vi "布尔与U8之间转换.vi"() -> ()   [LabVIEW 2023]
doc: "本VI是为《我和LabVIEW》一书编写的示例。\n关于本书的介绍请参考网页：\nhttp://ruanqizhen.spaces.live.com/blog/cns!5852D4F797C53FB6!4310.entry"
panel:
  out "*(类型 *) &x 2":u8
  out "*(类型 *) &x":bool
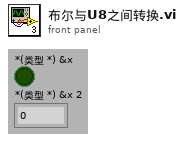
[diagram p1: front panel]
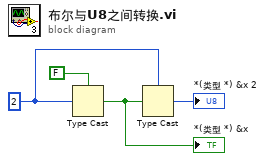
[diagram p0: block diagram]
diagram:
  w2 = u8 2 ("数值")
  n1 = Type Cast(type=FALSE, x=w2) -> (*(type *) &x=w3:bool)
  "*(类型 *) &x" <- w3
  n2 = Type Cast(type=w2, x=w3) -> (*(type *) &x=→"*(类型 *) &x 2":u8)
